vi "RequiredForAll-Mode.vi"(8 "error in (no error)":errorcluster, 11 "Class-Interface in":refnum<class "Class-Interface.lvclass">) -> (0 "error out":errorcluster, 2 "Mode":T1=enum."LabVIEW(DriverLayer)", 3 "Class-Interface out":refnum<class "Class-Interface.lvclass">)   [LabVIEW 2019, in "CAN-Interface.lvlib" / "Class-Interface.lvclass"]
uses:
  Class-Interface.lvclass
  <vilib>/lvAPT/.lib/HAL-Interface.lvlibp/HALInterface/Typedef/Def-Mode.ctl
  <vilib>/lvAPT/.lib/HAL-Interface.lvlibp/HALInterface/HALInterface.lvclass
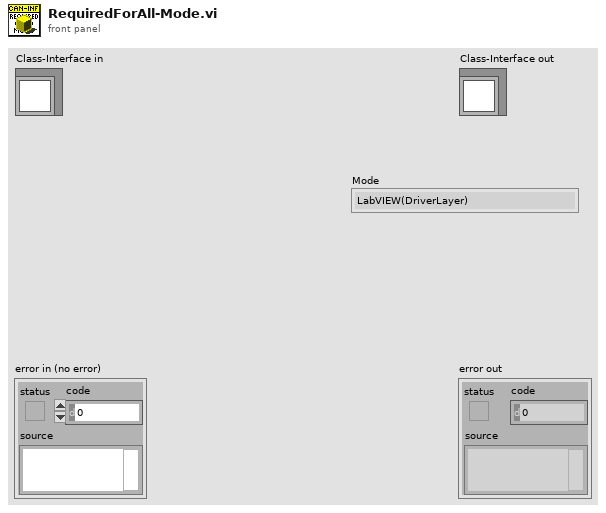
[diagram p1: front panel]
types:
  T1 = typedef "HAL-Interface.lvlibp/HALInterface.lvclass/Def-Mode.ctl" = enum16{"AbstractLayer", "LabVIEW(DriverLayer)", "DLL(DriverLayer)", "RPC(DriverLayer)"}
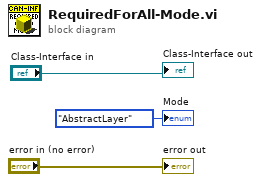
[diagram p0: block diagram]
diagram:
  "error out" <- "error in (no error)"
  "Class-Interface out" <- "Class-Interface in"
  "Mode" <- Def-Mode."AbstractLayer" ("Mode")
